vi "TDMSbuffersize.vi"(8 "error in (no error)":errorcluster, 10 "group names":string[](array[string]), 11 "Data Value Reference in":refnum<k34>) -> (0 "error out":errorcluster, 3 "Data Value Reference out":refnum<k34>)   [LabVIEW 2020]
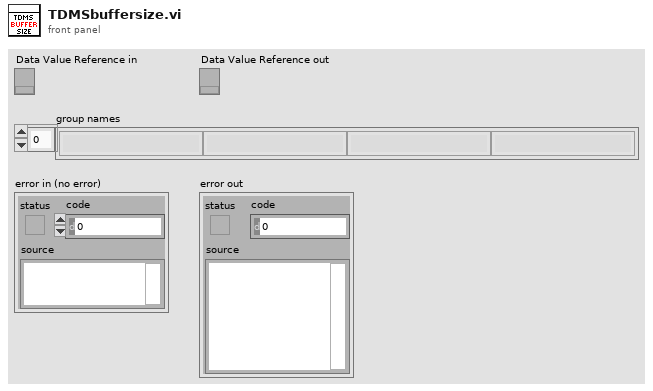
[diagram p1: front panel]
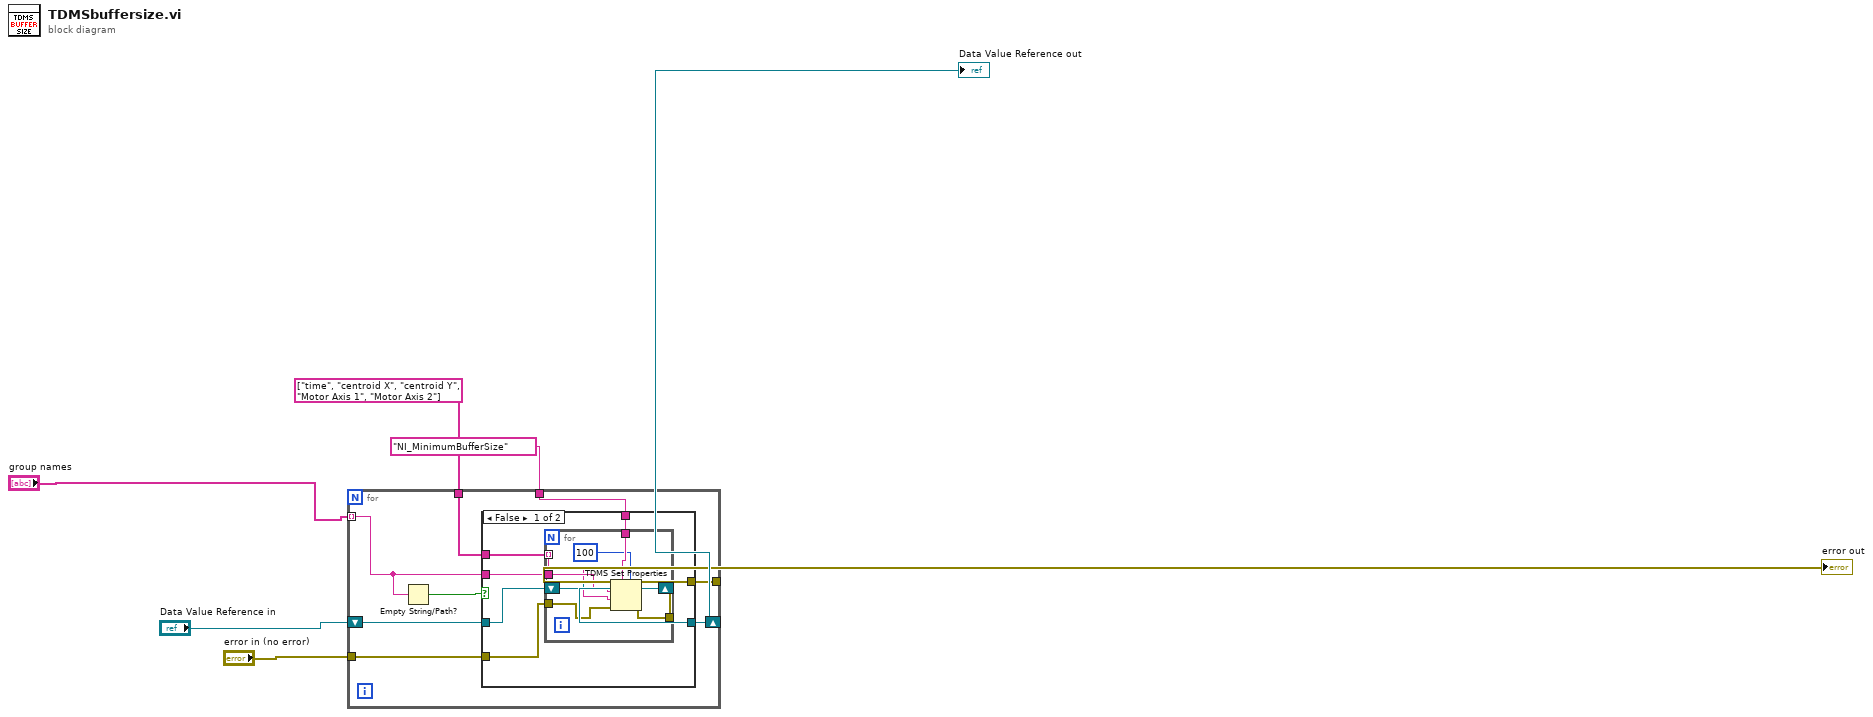
[diagram p0: block diagram]
diagram:
  n1 = for {
    tunnel: "error in (no error)" -> [w14]
    tunnel: [w13] -> w4
    tunnel: "group names" -> [w9] mode=indexing
    tunnel: "NI_MinimumBufferSize" -> [w12]
    shift-right: [w11] -> w7
    shift-left: "Data Value Reference in" -> [w15]
    tunnel: string[] ["time", "centroid X", "centroid Y", "Motor Axis 1", "Motor Axis 2"] ("appended array") -> [w10]
    n2 = Empty String/Path?(string/path=w9) -> (empty?=w8:bool)
    n3 = case shown="False" w8 {
      tunnel: w15 -> [w22 w32]
      tunnel: w14 -> [w21 w31]
      tunnel: [w20 w31] -> w13
      tunnel: w12 -> [w19 _]
      tunnel: [w18 w32] -> w11
      tunnel: w10 -> [w17 _]
      tunnel: w9 -> [w16 _]
      frame False {
        n4 = for {
          tunnel: w21 -> [w30]
          tunnel: w17 -> [w23] mode=indexing
          tunnel: [w29] -> w20
          tunnel: w16 -> [w28]
          tunnel: w19 -> [w26]
          shift-right: [w24] -> w18
          shift-left: w22 -> [w27]
          n5 = TDMS Set Properties(5:100, 7:w26, 8:w30, 9:w23, 10:w28, 11:w27) -> (0:w29:errorcluster, 3:w24:refnum<k34>)  [unwired: 2 out]
        }
      }
      frame True {
      }
    }
  }
  "Data Value Reference out" <- w7
  "error out" <- w4
